vi "Find All ProjectItems.vi"(8 "error in":errorcluster, 10 "ProjectItem type":string, 11 "ProjectItem refnum":refnum<vi>) -> (0 "error out":errorcluster, 3 "ProjectItems":cluster{"Path":path, "Display Name":string}[](array[cluster]))   [LabVIEW 2019]
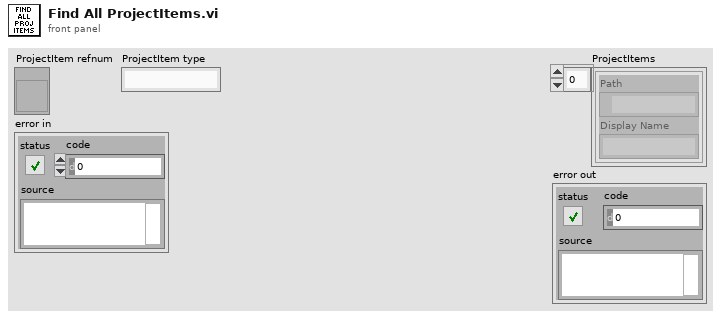
[diagram p1: front panel]
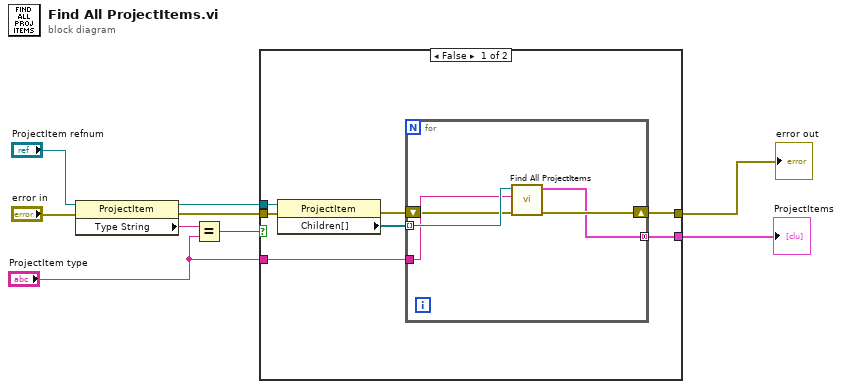
[diagram p0: block diagram]
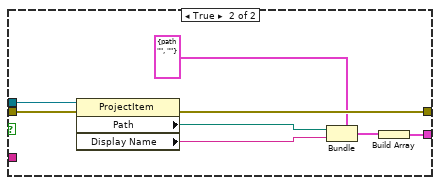
[diagram p2: hidden frame]
diagram:
  n1 = property class="ProjectItem"(reference="ProjectItem refnum", error in="error in") -> (reference out=w4:refnum<vi>, error out=w5:errorcluster, "Type String"=w7:string)
  n2 = Equal?(x=w7, y="ProjectItem type") -> (x = y?=w6:bool)
  n3 = case shown="False" w6 {
    tunnel: w5 -> [w13 w29]
    tunnel: w4 -> [w14 w28]
    tunnel: [w11 w27] -> w2
    tunnel: [w10 w22] -> w3
    tunnel: "ProjectItem type" -> [w12 _]
    frame False {
      n4 = property class="ProjectItem"(reference=w14, error in=w13) -> (error out=w16:errorcluster, "Children[]"=w15:refnum<vi>[])  [unwired: 1 out]
      n5 = for {
        tunnel: w15 -> [w21] mode=indexing
        tunnel: w12 -> [w20]
        shift-right: [w18] -> w11
        shift-left: w16 -> [w19]
        tunnel: [w17] -> w10 mode=concatenating
        n6 = call "Find All ProjectItems.vi"("error in"=w19, "ProjectItem type"=w20, "ProjectItem refnum"=w21) -> ("error out"=w18:errorcluster, "ProjectItems"=w17:cluster{"Path":path, "Display Name":string}[])  [unwired: 7 in]
      }
    }
    frame True {
      n7 = property class="ProjectItem"(reference=w28, error in=w29) -> (error out=w27:errorcluster, "Path"=w26:path, "Display Name"=w25:string)  [unwired: 1 out]
      n8 = Bundle(cluster=cluster{"Path":path, "Display Name":string} {"Path"=path "", "Display Name"=""}, "Path"=w26, "Display Name"=w25) -> (w23:cluster{"Path":path, "Display Name":string})
      n9 = Build Array(w23) -> (w22:cluster{"Path":path, "Display Name":string}[])
    }
  }
  "ProjectItems" <- w3
  "error out" <- w2
